vi "single sweep - upload freq window.vi"(4 "first time ?":bool=TRUE, 6 "timeout":dbl, 8 "error in (no error)":errorcluster, 9 "F-window array":dbl[](array[numeric]), 10 "task in":refnum<k21>, 11 "RUS settings":T1={"NI-DAQ lockin settings"={"Samples per sine wave"=0, "Sine waves per freq step"=0, "Output Representation"=enum."Real/Imaginary", "Low-pass filter"=enum."Butterworth", "Ranges and couplings "=[]}, "Fast swep settings"={"Update rate (Hz)"=250.0, "Start F, Hz"=200000.0, "Stop F"=1700000.0, "Number of points"=30000, "Amplitude"=2.1, "Init&amplitude"=TRUE, "IF"=1000.0, "Time constant"=0.1}, "Pre-sweep delay, s"=0.0, "Lockin mode"=enum."NI-DAQ", "SR Lockin"="GPIB0::10::INSTR", "DAQmx Device"="Dev3", "Clock Multiplier"=64, "Fast Sweep Data Out"={"DO clock task"="", "DO task"="", "Update clock task"="", "DAQ lockin task"="", "Pre-sweep counter task"=""}, "Lockin Range, V"=0.0, "F Array"=[], "Freq. update clock terminal"="", "DO Clock Rate (Hz)"=5000000.0, "ADC clock terminal"="/PFI4", "Pre-sweep counter terminal"="/PFI4", "Samples per read"=10, "DO clock terminal"="", "Pre-sweep points"=0, "F points per write"=0, "Total sweep time, s"=1000.0, "Initial SYNTH phase"=0.0, "Record IF"=FALSE, "Save data settings"={"Save data"=TRUE, "Data Root Path"=path "", "File Prefix"="", "File Format"=enum."ASCII", "Save column names"=TRUE, "File Comments"="<Description of the current file>", "User/Prj"="<User Name/Project Description>"}, "Data file path"=path "", "New data user event"=refnum, "Stop user event"=refnum, "Number of channels"=1, "Auto-phase"=FALSE} {"Lockin Range, V" format="%#_6e"; "Fast swep settings"."IF" format="%#_6p"; "Fast swep settings"."Amplitude" min=0.0 max=2.5; "Fast swep settings"."Number of points" format="%.0p"; "Fast swep settings"."Stop F" format="%#_6p"; "Fast swep settings"."Start F, Hz" format="%#_6p"; "Fast swep settings"."Update rate (Hz)" format="%0.2f"; "NI-DAQ lockin settings"."Ranges and couplings"."Coupling" items=["default"=-1, "RSE"=10083, "NRSE"=10078, "Differential"=10106, "Pseudodifferential"=12529]}) -> (0 "error out":errorcluster, 2 "task out":refnum<k21>, 3 "RUS settings out":T1={"NI-DAQ lockin settings"={"Samples per sine wave"=0, "Sine waves per freq step"=0, "Output Representation"=enum."Real/Imaginary", "Low-pass filter"=enum."Butterworth", "Ranges and couplings "=[]}, "Fast swep settings"={"Update rate (Hz)"=250.0, "Start F, Hz"=200000.0, "Stop F"=1700000.0, "Number of points"=30000, "Amplitude"=2.1, "Init&amplitude"=TRUE, "IF"=1000.0, "Time constant"=0.1}, "Pre-sweep delay, s"=0.0, "Lockin mode"=enum."NI-DAQ", "SR Lockin"="GPIB0::10::INSTR", "DAQmx Device"="Dev3", "Clock Multiplier"=64, "Fast Sweep Data Out"={"DO clock task"="", "DO task"="", "Update clock task"="", "DAQ lockin task"="", "Pre-sweep counter task"=""}, "Lockin Range, V"=0.0, "F Array"=[], "Freq. update clock terminal"="", "DO Clock Rate (Hz)"=5000000.0, "ADC clock terminal"="/PFI4", "Pre-sweep counter terminal"="/PFI4", "Samples per read"=10, "DO clock terminal"="", "Pre-sweep points"=0, "F points per write"=0, "Total sweep time, s"=1000.0, "Initial SYNTH phase"=0.0, "Record IF"=FALSE, "Save data settings"={"Save data"=TRUE, "Data Root Path"=path "", "File Prefix"="", "File Format"=enum."ASCII", "Save column names"=TRUE, "File Comments"="<Description of the current file>", "User/Prj"="<User Name/Project Description>"}, "Data file path"=path "", "New data user event"=refnum, "Stop user event"=refnum, "Number of channels"=1, "Auto-phase"=FALSE} {"Lockin Range, V" format="%#_6e"; "Fast swep settings"."IF" format="%#_6p"; "Fast swep settings"."Amplitude" min=0.0 max=2.5; "Fast swep settings"."Number of points" format="%.0p"; "Fast swep settings"."Stop F" format="%#_6p"; "Fast swep settings"."Start F, Hz" format="%#_6p"; "Fast swep settings"."Update rate (Hz)" format="%0.2f"; "NI-DAQ lockin settings"."Ranges and couplings"."Coupling" items=["default"=-1, "RSE"=10083, "NRSE"=10078, "Differential"=10106, "Pseudodifferential"=12529]}, 5 "DO array  making time":u32, 7 "DO write time":u32)   [LabVIEW 2015]
uses:
  Libraries/RUS/Controls/RUS settings.ctl
  Libraries/RUS/Controls/RUS NI-DAQ Lockin Settings.ctl
  Libraries/RUS/Controls/Sweep settings.ctl
  DAQ/Libraries/File/Controls/Save data settings.ctl
  DAQ/Libraries/File/Controls/File formats.ctl
  <vilib>/DAQmx/write.llb/DAQmx Write (Digital 1D U32 1Chan NSamp).vi
  <vilib>/DAQmx/miscellaneous.llb/DAQmx Fill In Error Info.vi
panel:
  in  "auto start":bool=TRUE
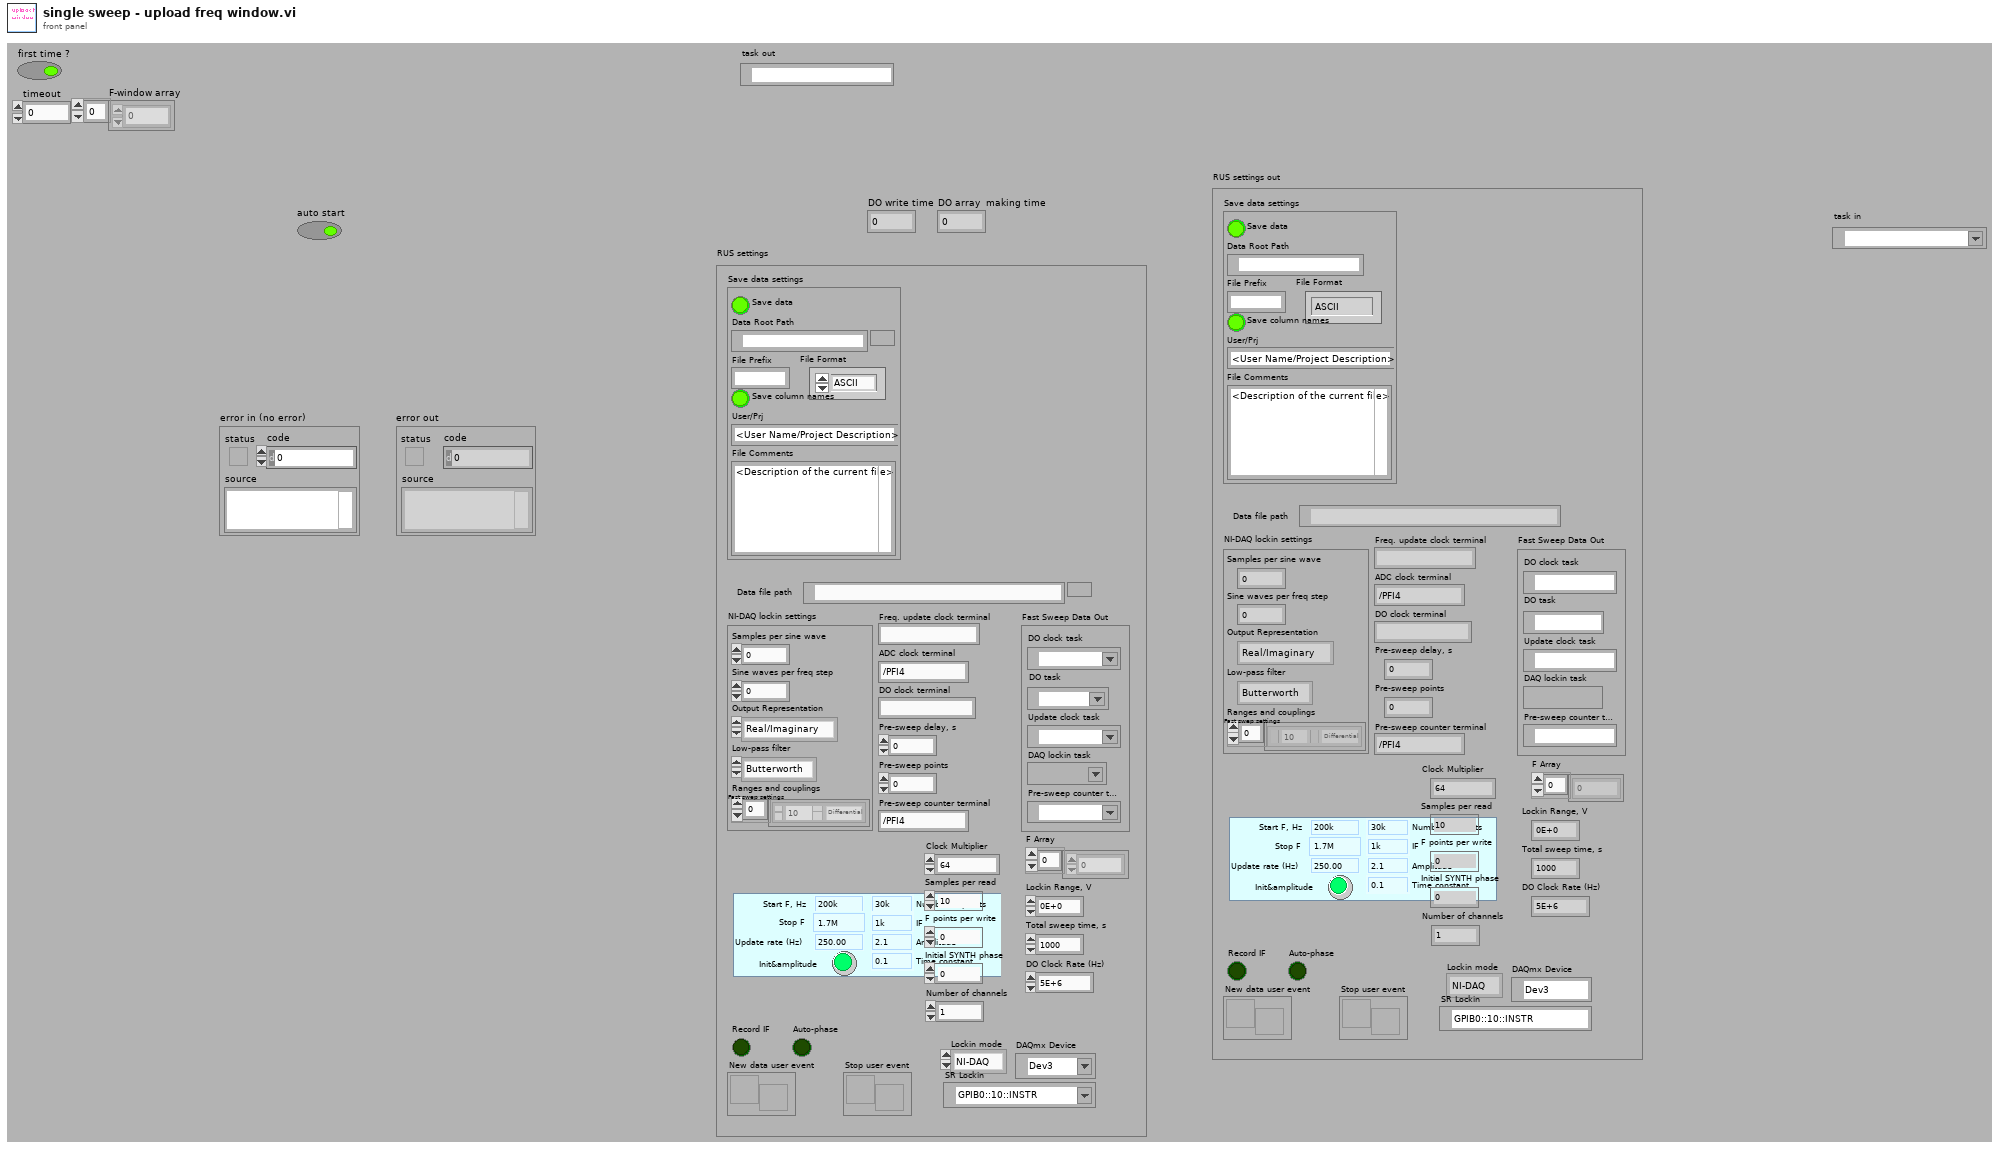
[diagram p1: front panel]
types:
  T1 = typedef "RUS settings.ctl" = cluster{"NI-DAQ lockin settings":T2, "Fast swep settings":T3, "Pre-sweep delay, s":dbl, "Lockin mode":enum16{"SRS", "NI-DAQ"}, "SR Lockin":refnum<visa-resource-name>, "DAQmx Device":tag, "Clock Multiplier":i32, "Fast Sweep Data Out":cluster{"DO clock task":refnum<k21>, "DO task":refnum<k21>, "Update clock task":refnum<k21>, "DAQ lockin task":refnum<k21>, "Pre-sweep counter task":refnum<k21>}, "Lockin Range, V":sgl, "F Array":dbl[], "Freq. update clock terminal":string, "DO Clock Rate (Hz)":dbl, "ADC clock terminal":string, "Pre-sweep counter terminal":string, "Samples per read":i32, "DO clock terminal":string, "Pre-sweep points":i32, "F points per write":i32, "Total sweep time, s":dbl, "Initial SYNTH phase":dbl, "Record IF":bool, "Save data settings":T4, "Data file path":path, "New data user event":refnum<user-event>, "Stop user event":refnum<user-event>, "Number of channels":i32, "Auto-phase":bool}
  T2 = typedef "RUS NI-DAQ Lockin Settings.ctl" = cluster{"Samples per sine wave":i32, "Sine waves per freq step":i32, "Output Representation":enum16{"Real/Imaginary", "Polar"}, "Low-pass filter":enum16{"No filtering", "Butterworth", "Bessel"}, "Ranges and couplings ":cluster{"Range":dbl, "Coupling":i32}[]}
  T3 = typedef "Sweep settings.ctl" = cluster{"Update rate (Hz)":dbl, "Start F, Hz":dbl, "Stop F":dbl, "Number of points":i32, "Amplitude":dbl, "Init&amplitude":bool, "IF":dbl, "Time constant":dbl}
  T4 = typedef "Save data settings.ctl" = cluster{"Save data":bool, "Data Root Path":path, "File Prefix":string, "File Format":T5, "Save column names":bool, "File Comments":string, "User/Prj":string}
  T5 = typedef "File formats.ctl" = enum16{"TDMS", "ASCII", "BINARY"}
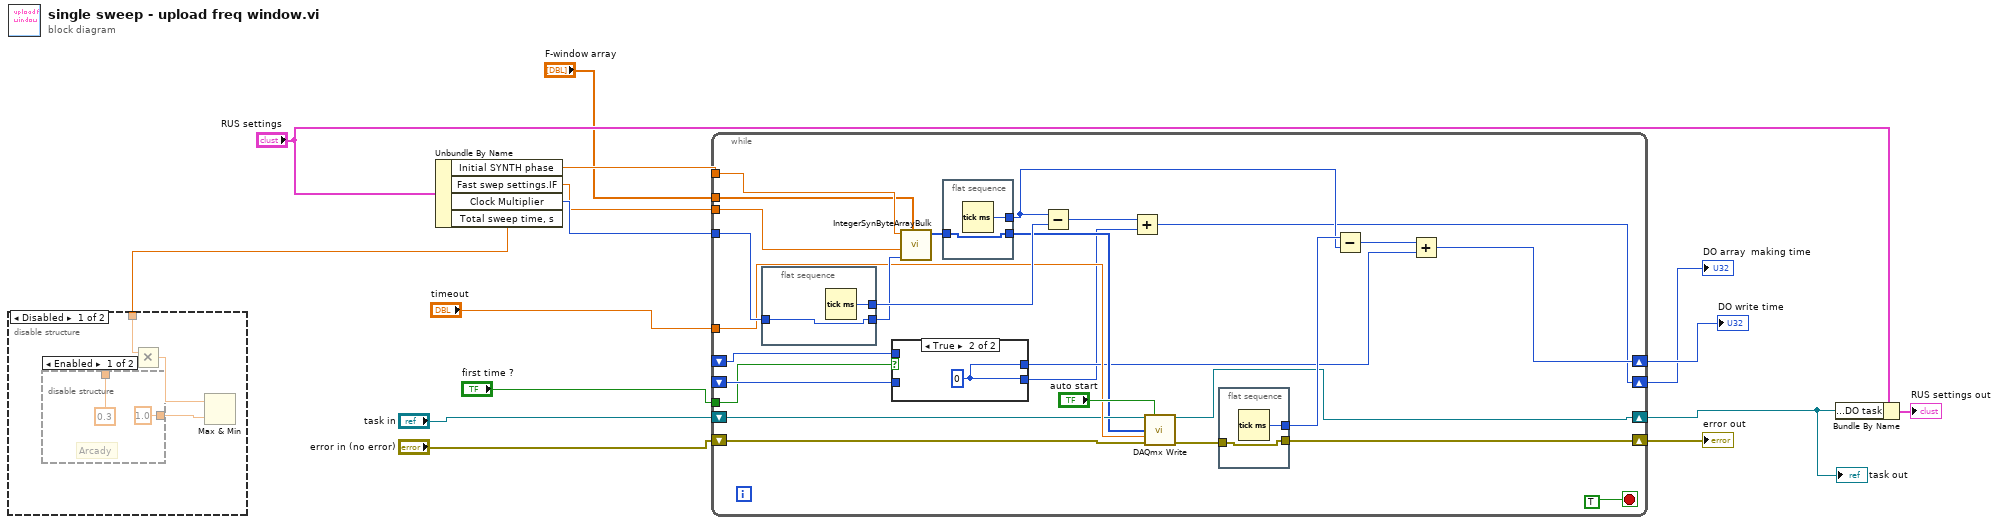
[diagram p0: block diagram]
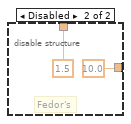
[diagram p3: hidden frame]
diagram:
  n1 = Unbundle By Name("RUS settings") -> ("Initial SYNTH phase"=w7:dbl, "Fast swep settings.IF"=w10:dbl, "Clock Multiplier"=w14:i32, "Total sweep time, s"=w8:dbl)
  n2 = disable-structure shown="Disabled" {
    disable-tunnel: w8 -> [w19 _]
    frame Disabled {
      n3 = disable-structure shown="Enabled" {
        disable-tunnel: [0.3 ("y") 1.5 ("y")] -> w17
        disable-tunnel: [1.0 ("y") 10.0 ("y")] -> w16
        frame Enabled {
          # "Arcady"
        }
        frame Disabled {
          # "Fedor's"
        }
      }
      n4 = Multiply(x=w19, y=w17) -> (x*y=w18:dbl)
      n5 = Max & Min(x=w18, y=w16) -> ()  [unwired: 2 out]
    }
    frame Enabled {
    }
  }
  n6 = while {
    tunnel: w14 -> [w49]
    tunnel: "F-window array" -> [w27]
    tunnel: w7 -> [w43]
    tunnel: w10 -> [w42]
    shift-right: [w25] -> w13
    shift-left: "error in (no error)" -> [w35]
    shift-right: [w26] -> w1
    shift-left: "task in" -> [w34]
    shift-right: [w38] -> w12
    shift-left: _ -> [w31]
    shift-right: [w37] -> w11
    shift-left: _ -> [w29]
    tunnel: "timeout" -> [w36]
    tunnel: "first time ?" -> [w28]
    stop <- TRUE stop-if-true
    n7 = flat-sequence {
      tunnel: [w59] -> w41
      tunnel: w49 -> [w59]
      tunnel: [w58] -> w45
      frame #0 {
        n8 = Tick Count (ms)() -> (millisecond timer value=w58:u32)
      }
    }
    n9 = case shown="True" w28 {
      tunnel: [w52 w53] -> w32
      tunnel: w31 -> [w52 _]
      tunnel: [w51 w53] -> w30
      tunnel: w29 -> [w51 _]
      frame False {
      }
      frame True {
        w53 = u32 0
      }
    }
    n10 = call "IntegerSynByteArrayBulk.vi"("Input  F1 array"=w27, "Clock multiplier"=w41, "Local Oscillator (IF,f2)"=w42, "Phase (degrees)"=w43) -> ("output array"=w40:u8[])  [unwired: 7 in]
    n11 = flat-sequence {
      tunnel: [w55] -> w33
      tunnel: w40 -> [w55]
      tunnel: [w54] -> w39
      frame #0 {
        n12 = Tick Count (ms)() -> (millisecond timer value=w54:u32)
      }
    }
    n13 = Subtract(x=w39, y=w45) -> (x-y=w44:u32)
    n14 = Add(x=w44, y=w30) -> (x+y=w37:u32)
    n15 = call-poly <vilib>:"DAQmx Write.vi"("task/channels in"=w34, "auto start"="auto start", "data"=w33, "timeout"=w36, "error in"=w35) -> ("task out"=w26:refnum<k21>, "error out"=w48:errorcluster)  [unwired: 9 out]
    n16 = flat-sequence {
      tunnel: [w57] -> w25
      tunnel: w48 -> [w57]
      tunnel: [w56] -> w47
      frame #0 {
        n17 = Tick Count (ms)() -> (millisecond timer value=w56:u32)
      }
    }
    n18 = Subtract(x=w47, y=w39) -> (x-y=w46:u32)
    n19 = Add(x=w46, y=w32) -> (x+y=w38:u32)
  }
  "error out" <- w13
  "DO write time" <- w12
  "DO array  making time" <- w11
  "task out" <- w1
  n20 = Bundle By Name(cluster="RUS settings", "Fast Sweep Data Out.DO task"=w1) -> (→"RUS settings out":T1)
